vi "Remove Driver Settings.vi"(8 "error in (no error)":errorcluster, 9 "Command Settings":refnum<class "CommandSetting.lvclass">[](array[class]), 10 "Command Id":string, 11 "Driver in":refnum<class "Driver.lvclass">) -> (0 "error out":errorcluster, 2 "Settings Removed":u32, 3 "Driver out":refnum<class "Driver.lvclass">)   [LabVIEW 2023, in "HAF.lvlib" / "Driver.lvclass"]
doc: "Removes the Driver Settings for the given Command Settings from the collection. The number removed is reported."
uses:
  Driver.lvclass
  Driver.lvclass/Driver.ctl
  CommandSetting/CommandSetting.lvclass
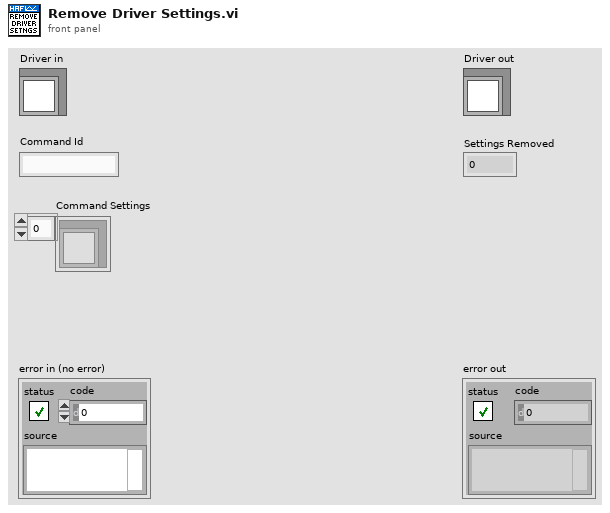
[diagram p1: front panel]
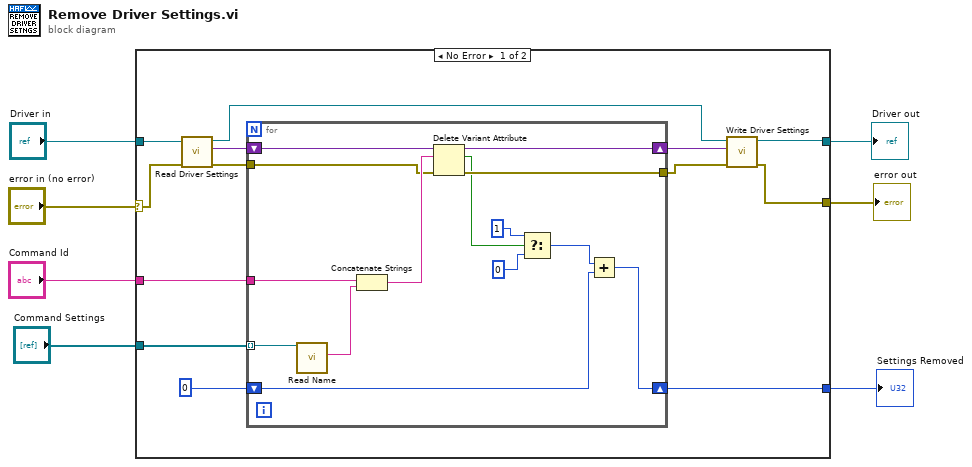
[diagram p0: block diagram]
diagram:
  n1 = case shown="No Error" "error in (no error)" {
    selector: "error in (no error)" -> [w19 w36]
    tunnel: [w9 w36] -> w6
    tunnel: [w10 w35] -> w4
    tunnel: "Driver in" -> [w20 w35]
    tunnel: "Command Id" -> [w16 _]
    tunnel: "Command Settings" -> [w15 _]
    tunnel: [w8 _] -> w1
    frame No Error {
      n2 = call-dynamic "Read Driver Settings.vi"("error in (no error)"=w19, "Driver in"=w20) -> ("error out"=w17:errorcluster, "Driver Settings"=w18:variant, "Driver out"=w12:refnum<class "Driver.lvclass">)  [unwired: 7 in]
      n3 = for {
        shift-right: [w28] -> w11
        shift-left: w18 -> [w31]
        tunnel: w17 -> [w29]
        tunnel: w16 -> [w33]
        tunnel: w15 -> [w34] mode=indexing
        shift-right: [w21] -> w8
        shift-left: u32 0 ("Removed Count") -> [w22]
        tunnel: [w27] -> w13
        n4 = call-dynamic "Read Name.vi"("Setting in"=w34) -> ("Name"=w32:string)  [unwired: 8 in, 2 out]
        n5 = Concatenate Strings(w33, w32) -> (w30:string)
        n6 = Delete Variant Attribute(4:w29, 6:w30, 7:w31) -> (0:w27:errorcluster, 2:w26:bool, 3:w28:variant)
        n7 = Select(t=u32 1, s=w26, f=u32 0) -> (s? t:f=w23:u32)
        n8 = Add(x=w23, y=w22) -> (x+y=w21:u32)
      }
      n9 = call-dynamic "Write Driver Settings.vi"("error in (no error)"=w13, "Driver Settings"=w11, "Driver in"=w12) -> ("error out"=w9:errorcluster, "Driver out"=w10:refnum<class "Driver.lvclass">)  [unwired: 7 in]
    }
    frame Error {
    }
  }
  "error out" <- w6
  "Driver out" <- w4
  "Settings Removed" <- w1
